vi "NP04_DSS_TRANSFORM Facq to tdms.vi"() -> ()   [LabVIEW 2017]
panel:
  in  "Path":path=path "F:/NP04/NP04_HV_test_Lab/FACQ files"
  out "In progress":i32(slide) scale=0.0..200000.0
  in  "File Type":enum16{"SD Facq", "FD Facq"}(ring)=enum."FD Facq"
  in  "Data Period":u16(ring)=1 items=["50 us"=1, "200 us"=4, "1 ms"=20, "10 ms"=200]
  out "# of data":i32
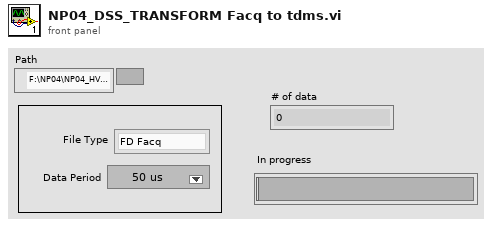
[diagram p1: front panel]
types:
  T1 = cluster{"Timestamp":timestamp, "timestamp ns":u64, "Acquired Values":sgl[], "Calculated Values":sgl[]}
  T2 = enum16{"open", "open or create", "create or replace", "create", "open (read-only)"}
  T3 = enum16{"big-endian, network order", "native, host order", "little-endian"}
  T4 = cluster{"Timestamp":timestamp, "timestamp ns":u64, "Acquired Values":sgl[], "Calculated Values":sgl[]}[]
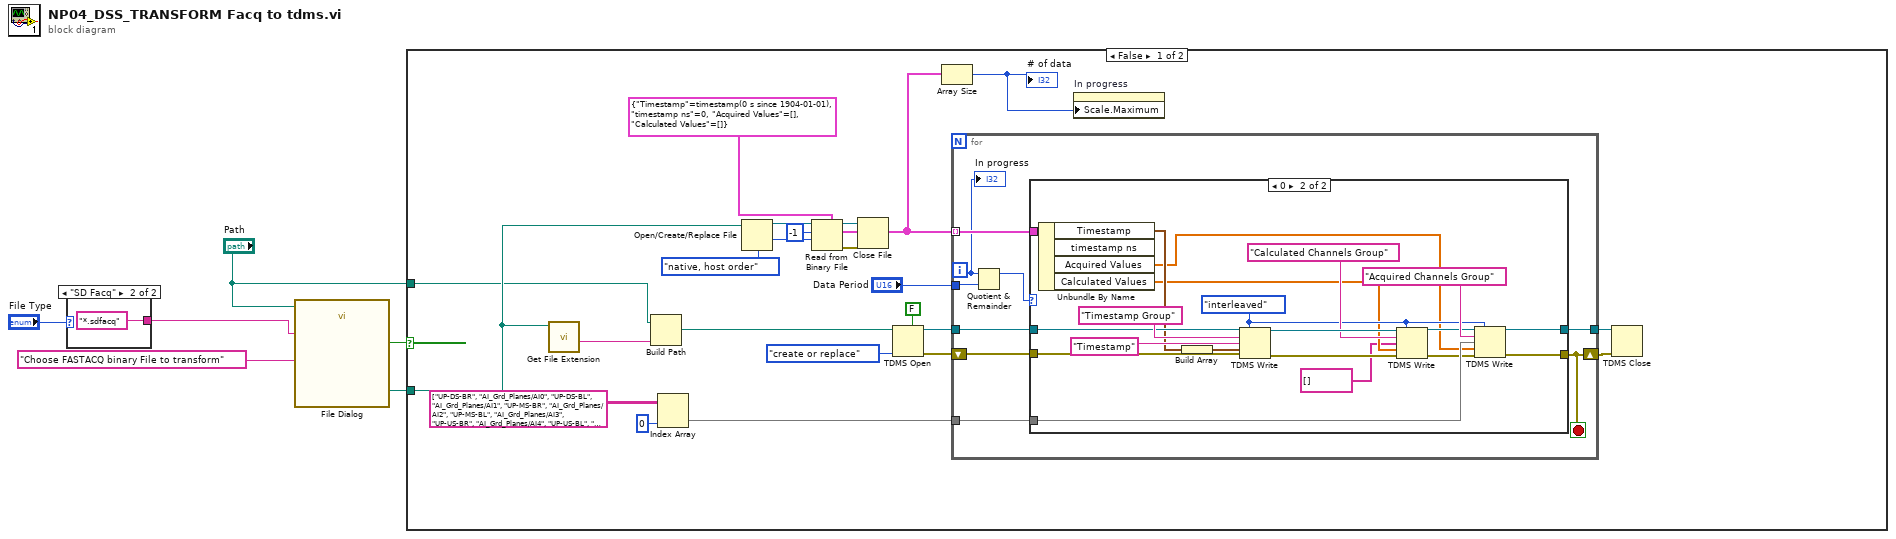
[diagram p0: block diagram]
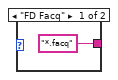
[diagram p2: hidden frame]
diagram:
  n1 = case shown="\"SD Facq\"" "File Type" {
    tunnel: ["*.facq" ("pattern (all files)") "*.sdfacq" ("pattern (all files)")] -> w1
    frame "FD Facq" {
    }
    frame "SD Facq" {
    }
  }
  n2 = call "File Dialog"("start path"="Path", "prompt"="Choose FASTACQ binary File to transform", "pattern (all files)"=w1) -> ("selected path"=w5:path, "cancelled"=w4:bool)  [unwired: 9 in, 2 out]
  n3 = case shown="False" w4 {
    tunnel: w5 -> [w20 _]
    tunnel: "Path" -> [w13 _]
    frame False {
      n4 = call <vilib>:"Get File Extension.vi"("file"=w20) -> ("filename without extension"=w19:string)  [unwired: 6 in, 4 out]
      n5 = Build Path(base path=w13, name or relative path=w19) -> (appended path=w18:path)
      n6 = Index Array(array=string[][] [["UP-DS-BR", "AI_Grd_Planes/AI0"], ["UP-DS-BL", "AI_Grd_Planes/AI1"], ["UP-MS-BR", "AI_Grd_Planes/AI2"], ["UP-MS-BL", "AI_Grd_Planes/AI3"], ["UP-US-BR", "AI_Grd_Planes/AI4"], ["UP-US-BL", "AI_Grd_Planes/AI5"], ["DN-DS-BR", "AI_Grd_Planes/AI6"], ["DN-DS-BL", "AI_Grd_Planes/AI7"], ["DN-MS-BR", "AI_Grd_Planes/AI16"], ["DN-MS-BL", "AI_Grd_Planes/AI17"], ["DN-US-BR", "AI_Grd_Planes/AI18"], ["DN-US-BL", "AI_Grd_Planes/AI19"], ["GND012", "AI_Grd_Planes/AI20"], ["GND013", "AI_Grd_Planes/AI21"], ["GND014", "AI_Grd_Planes/AI22"], ["LAr_Lvl", "AI_Grd_Planes/AI23"], ["HV_Trip_Current", "Virtual Channel"], ["DSS_ Digital_Outputs", ""]] ("Al_HI channels"), index (col)=0) -> (element=w10:string[])  [unwired: 1 in]
      n7 = Open/Create/Replace File(file path (use dialog)=w20) -> (refnum out=w30:refnum<file>)  [unwired: 5 in, 2 out]
      n8 = Read from Binary File(5:T1 {"Timestamp"=timestamp(0 s since 1904-01-01), "timestamp ns"=0, "Acquired Values"=[], "Calculated Values"=[]}, 9:T3."native, host order" ("byte order (0:big-endian, network order)"), 10:-1 ("count (1)"), 11:w30) -> (0:w23:errorcluster, 2:w17:T4, 3:w22:refnum<file>)  [unwired: 2 in, 1 out]
      n9 = Close File(refnum=w22, error in=w23) -> ()  [unwired: 2 out]
      n10 = TDMS Open(5:FALSE ("create index file? (T)"), 10:T2."create or replace" ("operation (0:open)"), 11:w18) -> (0:w15:errorcluster, 3:w26:refnum<k34>)  [unwired: 4 in]
      n11 = Array Size(array=w17) -> (size(s)=w9:i32)
      "# of data" <- w9
      n12 = for {
        tunnel: w17 -> [w39] mode=indexing
        tunnel: w26 -> [w38]
        tunnel: w10 -> [w37]
        tunnel: [w36] -> w24
        shift-right: [w34] -> w14
        shift-left: w15 -> [w35]
        tunnel: "Data Period" -> [w33]
        i -> [w31]
        stop <- w34 stop-if-true
        n13 = Quotient & Remainder(x=w31, y=w33) -> (x-y*floor(x/y)=w32:i32)  [unwired: 1 out]
        n14 = case shown="0" w32 {
          tunnel: w39 -> [_ w61]
          tunnel: w38 -> [w41 w52]
          tunnel: w37 -> [_ w50]
          tunnel: [w41 w47] -> w36
          tunnel: w35 -> [w40 w46]
          tunnel: [w40 w43] -> w34
          frame 1, Default {
          }
          frame 0 {
            w54 = enum16{"decimated", "interleaved"}."interleaved" ("data layout (0:decimated)")
            n15 = Unbundle By Name(w61) -> ("Timestamp"=w51:timestamp, "Acquired Values"=w48:sgl[], "Calculated Values"=w49:sgl[])  [unwired: 1 out]
            n16 = Build Array(w51) -> (w60:timestamp[])
            n17 = TDMS Write(0:w52, 1:w54, 5:"Timestamp Group", 7:"Timestamp", 9:w60, 11:w46) -> (4:w58:refnum<k34>, 15:w45:errorcluster)  [unwired: 2 out]
            n18 = TDMS Write(0:w58, 1:w54, 5:"Calculated Channels Group", 7:string[] [] ("channel name(s) in (Untitled)"), 9:w49, 11:w45) -> (4:w55:refnum<k34>, 15:w44:errorcluster)  [unwired: 2 out]
            n19 = TDMS Write(0:w55, 1:w54, 5:"Acquired Channels Group", 7:w50, 9:w48, 11:w44) -> (4:w47:refnum<k34>, 15:w43:errorcluster)  [unwired: 2 out]
          }
        }
        "In progress" <- w31
      }
      n20 = property on="In progress" class="Slide (strict)"("Scale.Maximum"=w9) -> ()  [unwired: 2 in, 2 out]
      n21 = TDMS Close(8:w14, 11:w24) -> ()  [unwired: 2 out]
    }
    frame True {
    }
  }
